vi "Store Controller Enqueuer.vi"(7 "State":enum16{"Write", "Read"}(ring)=enum."Read", 11 "Controller Enqueuer In":refnum<class "Message Enqueuer.lvclass">) -> (3 "Controller Enqueuer Out":refnum<class "Message Enqueuer.lvclass">)   [LabVIEW 2017, in "Controller.lvlib" / "gController.lvclass"]
uses:
  gController.lvclass
  <vilib>/ActorFramework/Message Enqueuer/Message Enqueuer.lvclass
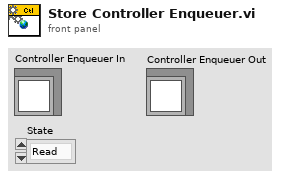
[diagram p1: front panel]
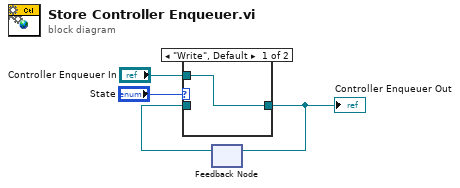
[diagram p0: block diagram]
diagram:
  n1 = feedback #1() -> (w1:refnum<class "Message Enqueuer.lvclass">)  [unwired: 1 in]
  n2 = case shown="\"Write\", Default" "State" {
    tunnel: "Controller Enqueuer In" -> [w5 _]
    tunnel: [w5 w6] -> w2
    tunnel: w1 -> [_ w6]
    frame "Write", Default {
    }
    frame "Read" {
    }
  }
  "Controller Enqueuer Out" <- w2
  n3 = feedback-in #1(w2) -> ()
